vi "GetParam.vi"(8 "error in (no error)":errorcluster caption="entrée d'erreur (pas d'erreur)", 11 "LeavePOut.lvclass":refnum<class "LeavePOut.lvclass">) -> (0 "error out":errorcluster caption="sortie d'erreur", 2 "LeavePOut":cluster{"p":i32}={"p"=2}, 3 "LeavePOut.lvclass":refnum<class "LeavePOut.lvclass">)   [LabVIEW 2020, in "LeavePOut.lvclass"]
doc: "Get Parameters"
uses:
  LeavePOut.lvclass
  LeavePOut.lvclass/LeavePOut.ctl
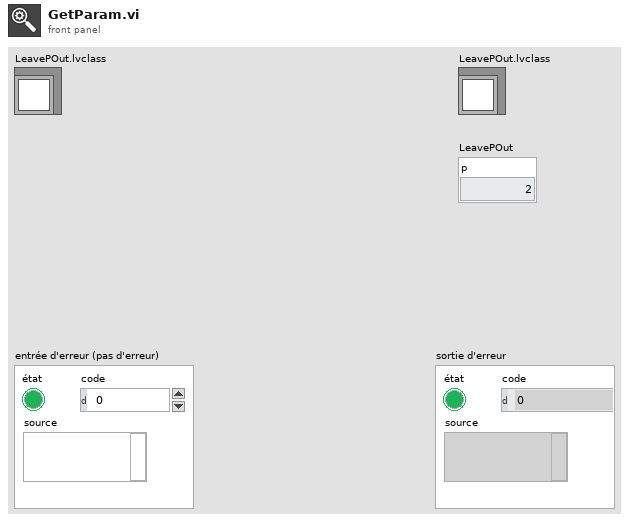
[diagram p1: front panel]
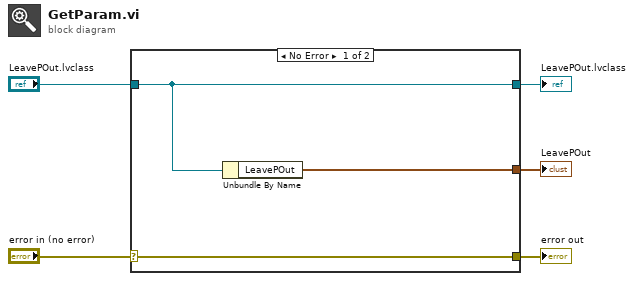
[diagram p0: block diagram]
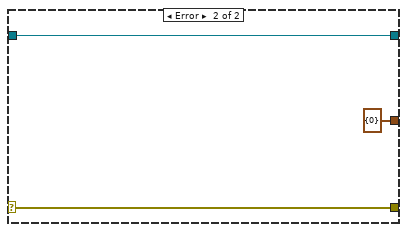
[diagram p2: hidden frame]
diagram:
  n1 = case shown="No Error" "error in (no error)" {
    selector: "error in (no error)" -> [w8 w10]
    tunnel: [w8 w10] -> w4
    tunnel: [w7 w11] -> w2
    tunnel: "LeavePOut.lvclass" -> [w7 w11]
    tunnel: [w6 cluster{"p":i32} {"p"=0} ("LeavePOut")] -> w1
    frame No Error {
      n2 = Unbundle By Name(w7) -> ("LeavePOut"=w6:cluster{"p":i32})
    }
    frame Error {
    }
  }
  "error out" <- w4
  "LeavePOut.lvclass" <- w2
  "LeavePOut" <- w1
